vi "After Launch Init Core.vi"(8 "error in (no error)":errorcluster, 11 "CS++DIM-Server in":refnum<class "CS++DIM-Server.lvclass">) -> (0 "error out":errorcluster, 3 "CS++DIM-Server out":refnum<class "CS++DIM-Server.lvclass">)   [LabVIEW 2016, in "CS++DIM-Server.lvlib" / "CS++DIM-Server.lvclass"]
doc: "Use <b>Pre Launch init.vi</b> method only for sanity checks that are supposed to prevent the actor from launching if they fail. Use <B>this</B> method instead to initialize unique resources that must be released during the <b>Stop Core.vi</b> method. A corresponding high priority message will become dispatched before the <B>Actor Framework.lvlib:Actor.lvclass.Actor Core.vi</b> is called.\n\n<b>Derived classed should call the parent methode first</b> and their own initialization code after.\n\nRefer also to the ongoing discussion at https://decibel.ni.com/content/message/57394#57394."
uses:
  CS++DIM-Server.lvclass
  C:/User/Brand/LVP/CSPP-Dev/Packages/CSPP_Core/Actors/CS++BaseActor/CS++BaseActor.lvclass
  C:/Program Files (x86)/National Instruments/LabVIEW 2016/vi.lib/ActorFramework/Actor/Actor.lvclass
  CSPP_Core/Actors/CS++BaseActor/CS++BaseActor.lvclass/CS++BaseActor.ctl
  CS++DIM-Server.lvclass/CS++DIM-Server.ctl
  CSPP_Core/Classes/CS++ProcessVariables/ProcessVariable/PV.lvclass
  DIMConnection/DIMConnection.lvclass
  C:/User/Brand/LVP/CSPP-Dev/Packages/CSPP_Core/Classes/CS++ProcessVariables/PVConnection/PVConnection.lvclass
  CSPP_Core/Classes/CS++ProcessVariables/ProcessVariable/PV.lvclass/PV.ctl
  CSPP_Core/Classes/CS++ProcessVariables/PVConnection/PVConnection.lvclass/PVConnection.ctl
  <vilib>/ActorFramework/Actor/Actor.lvclass/Actor.ctl
  <vilib>/ActorFramework/Message Enqueuer/Message Enqueuer.lvclass/Message Enqueuer.ctl
  CSPP_Core/Actors/CS++BaseActor/Read Object Name.vi
  <vilib>/ActorFramework/Message Enqueuer/Init from Existing Queue.vi
  <vilib>/ActorFramework/Message Enqueuer/Enqueue.vi
  <vilib>/Utility/error.llb/Error Cluster From Error Code.vi
  <vilib>/ActorFramework/Message Priority Queue/Priority Enqueue.vi
  CSPP_Core/Actors/CS++BaseActor/CS++BaseActor.lvclass
  <vilib>/ActorFramework/Message Enqueuer/Message Enqueuer.lvclass
  <vilib>/ActorFramework/Message/Message.lvclass
  CSPP_Core/Classes/CS++ProcessVariables/PVConnection/PVConnection.lvclass
  CS++DIM-Server Messages/Publish Services Msg/Publish Services Msg.lvclass
  <vilib>/ActorFramework/Actor/Actor.lvclass
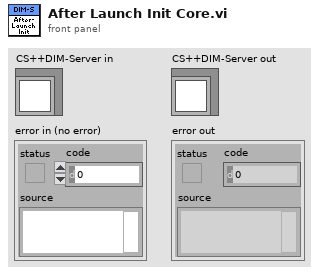
[diagram p1: front panel]
types:
  T1 = cluster{"Write Access":enum8{"Allowed", "Required", "None"}, "Read Access":enum8{"Allowed", "Required", "None"}}
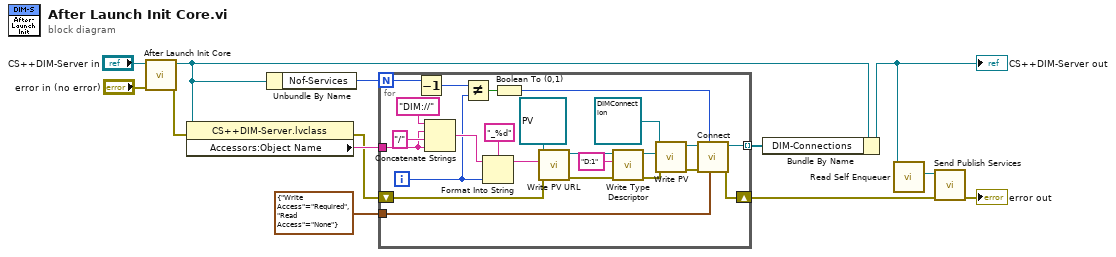
[diagram p0: block diagram]
diagram:
  n1 = call-parent "After Launch Init Core.vi"("error in (no error)"="error in (no error)", "CS++BaseActor in"="CS++DIM-Server in") -> ("error out"=w11:errorcluster, "CS++BaseActor out"=w5:refnum<class "CS++DIM-Server.lvclass">)  [unwired: 8 in]
  n2 = property class="CS++DIM-Server.lvclass"(reference=w5, error in=w11) -> (error out=w8:errorcluster, "Accessors:Object Name"=w10:string)  [unwired: 1 out]
  n3 = Unbundle By Name(w5) -> ("Nof-Services"=w9:i32)
  n4 = for {
    N: w9 -> [w18]
    tunnel: w10 -> [w36]
    shift-right: [w23] -> w2
    shift-left: w8 -> [w33]
    tunnel: T1 {"Write Access"=enum."Required", "Read Access"=enum."None"} ("Access (R/W allowed)") -> [w24]
    tunnel: [w22] -> w6 mode=indexing
    i -> [w16]
    n5 = Decrement(x=w18) -> (x-1=w17:i32)
    n6 = Concatenate Strings("DIM://", w36, "/" ("string"), w36) -> (w21:string)
    n7 = Not Equal?(x=w17, y=w16) -> (x != y?=w15:bool)
    n8 = Format Into String(format string="_%d", initial string=w21, w16) -> (resulting string=w19:string)  [unwired: 1 in, 1 out]
    n9 = Boolean To (0,1)(Boolean=w15) -> (0, 1=w14:i16)
    n10 = call "Write PV URL.vi"("error in (no error)"=w33, "PV URL"=w19, "PV in"=refnum<class "PV.lvclass"> refnum ("CS++ProcessVariables.lvlib:PV.lvclass")) -> ("error out"=w31:errorcluster, "PV out"=w32:refnum<class "PV.lvclass">)  [unwired: 7 in]
    n11 = call "Write Type Descriptor.vi"("error in (no error)"=w31, "Type Descriptor"="D:1", "PV in"=w32) -> ("error out"=w25:errorcluster, "PV out"=w29:refnum<class "PV.lvclass">)  [unwired: 7 in]
    n12 = call "Write PV.vi"("error in (no error)"=w25, "PV"=w29, "PVConnection in"=refnum<class "DIMConnection.lvclass"> refnum ("CS++DIM.lvlib:DIMConnection.lvclass")) -> ("error out"=w28:errorcluster, "PVConnection out"=w26:refnum<class "DIMConnection.lvclass">)  [unwired: 7 in]
    n13 = call "Connect.vi"("Access (R/W allowed)"=w24, "Mode (buffer)"=w14, "Error In"=w28, "PVConnection in"=w26) -> ("Error Out"=w23:errorcluster, "PVConnection out"=w22:refnum<class "DIMConnection.lvclass">)  [unwired: 6 in]
  }
  n14 = Bundle By Name(cluster=w5, "DIM-Connections"=w6) -> (w4:refnum<class "CS++DIM-Server.lvclass">)
  "CS++DIM-Server out" <- w4
  n15 = call <vilib>:"Read Self Enqueuer.vi"("Actor"=w4) -> ("Self Enqueuer"=w3:refnum<class "Message Enqueuer.lvclass">)  [unwired: 10 in]
  n16 = call "Send Publish Services.vi"("error in (no error)"=w2, "Message Enqueuer"=w3) -> ("error out"=→"error out":errorcluster)  [unwired: 8 in, 1 out]
